vi "FilterSingle.vi"(9 "Error in":errorcluster, 10 "Code to filter":i32) -> (1 "Error out":errorcluster, 2 "Code filtered?":bool)   [LabVIEW 2017, in "GPError.lvlib"]
doc: "Clears the error or warning on <B>Error in</B> if Code in <B>Error in</B> matches <B>Code to filter</B>.\n\nThis VI supports filtering appended errors, in which case it clears only those elements in the appended error collection that matches <B>Code to filter</B>.\n\n<B>Code filtered?</B> will be True only if <B>Error in</B> was filtered.\n\nThis VI is inlined.\n\nSteen Schmidt\nGPower\n18/7 2013"
uses:
  GPError.lvlib
panel:
  # "Copyright © 2013\nSteen Schmidt, GPower\nSee enclosed license file for terms and conditions"
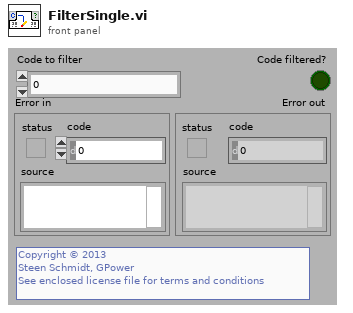
[diagram p1: front panel]
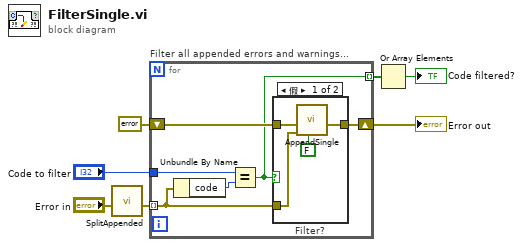
[diagram p0: block diagram]
diagram:
  n1 = call "SplitAppended.vi"("Appended errors in"="Error in") -> ("Errors out"=w6:errorcluster[])  [unwired: 10 in]
  n2 = for "Filter all appended errors and warnings..." {
    tunnel: w6 -> [w10] mode=indexing
    tunnel: "Code to filter" -> [w12]
    shift-right: [w9] -> w3
    shift-left: errorcluster {"status"=FALSE, "code"=0, "source"=""} ("error out") -> [w11]
    tunnel: [w8] -> w2 mode=indexing
    n3 = Unbundle By Name(w10) -> ("code"=w13:i32)
    n4 = Equal?(x=w12, y=w13) -> (x = y?=w8:bool)
    n5 = case "Filter?" shown="假" w8 {
      tunnel: w11 -> [w17 w18]
      tunnel: w10 -> [w16 _]
      tunnel: [w15 w18] -> w9
      frame False {
        n6 = call "AppendSingle.vi"("Only append if new?"=FALSE, "Error to append"=w16, "Error in"=w17) -> ("Appended errors out"=w15:errorcluster)  [unwired: 8 in]
      }
      frame True {
      }
    }
  }
  "Error out" <- w3
  n7 = Or Array Elements(Boolean array=w2) -> (logical OR=→"Code filtered?":bool)
